vi "Power Driver.vi"(0 "P CH0_curlim, A":dbl=0.08 min=0.01 max=1.0 format="%_6p", 1 "P CH0, V":dbl=3.3000000000000003 min=0.0 max=6.0 format="%_6p", 2 "P CH1_curlim, A":dbl=0.1 min=0.01 max=1.0 format="%_6p", 3 "P CH1_cur, A":dbl=2.0 min=0.0 max=20.0 format="%_6p", 4 "P CH2_curlim, A":dbl=0.01 min=0.01 max=1.0 format="%_6p", 5 "P CH2, V":dbl=-5.0 min=-20.0 max=0.0 format="%_6p", 6 "P CH0":bool, 7 "Instrument Handle In":refnum<k15>, 8 "P CH1":bool, 9 "Error In":errorcluster, 10 "P CH2":bool, 12 "Power OFF":bool) -> (11 "Error Out":errorcluster, 13 "Instrument Handle Out":refnum<k15>, 14 "P CH0_char":dbl(graph)=8.200132019086688e-05, 15 "P CH0_cur, A":dbl=8.200132019086688e-05 format="%_6g", 16 "P CH1_char":dbl(graph)=9.464711192498274e-07, 17 "P CH1_cur, A":dbl=9.464711192498274e-07 format="%_6g", 18 "P CH2_char":dbl(graph)=1.4003158139382402e-06, 19 "P CH2_cur, A":dbl=1.4003158139382402e-06 format="%_6g")   [LabVIEW 2018]
uses:
  <instrlib>/niDCPower/nidcpower.llb/niDCPower Measurement Type.ctl
panel:
  out "Power OFF":bool
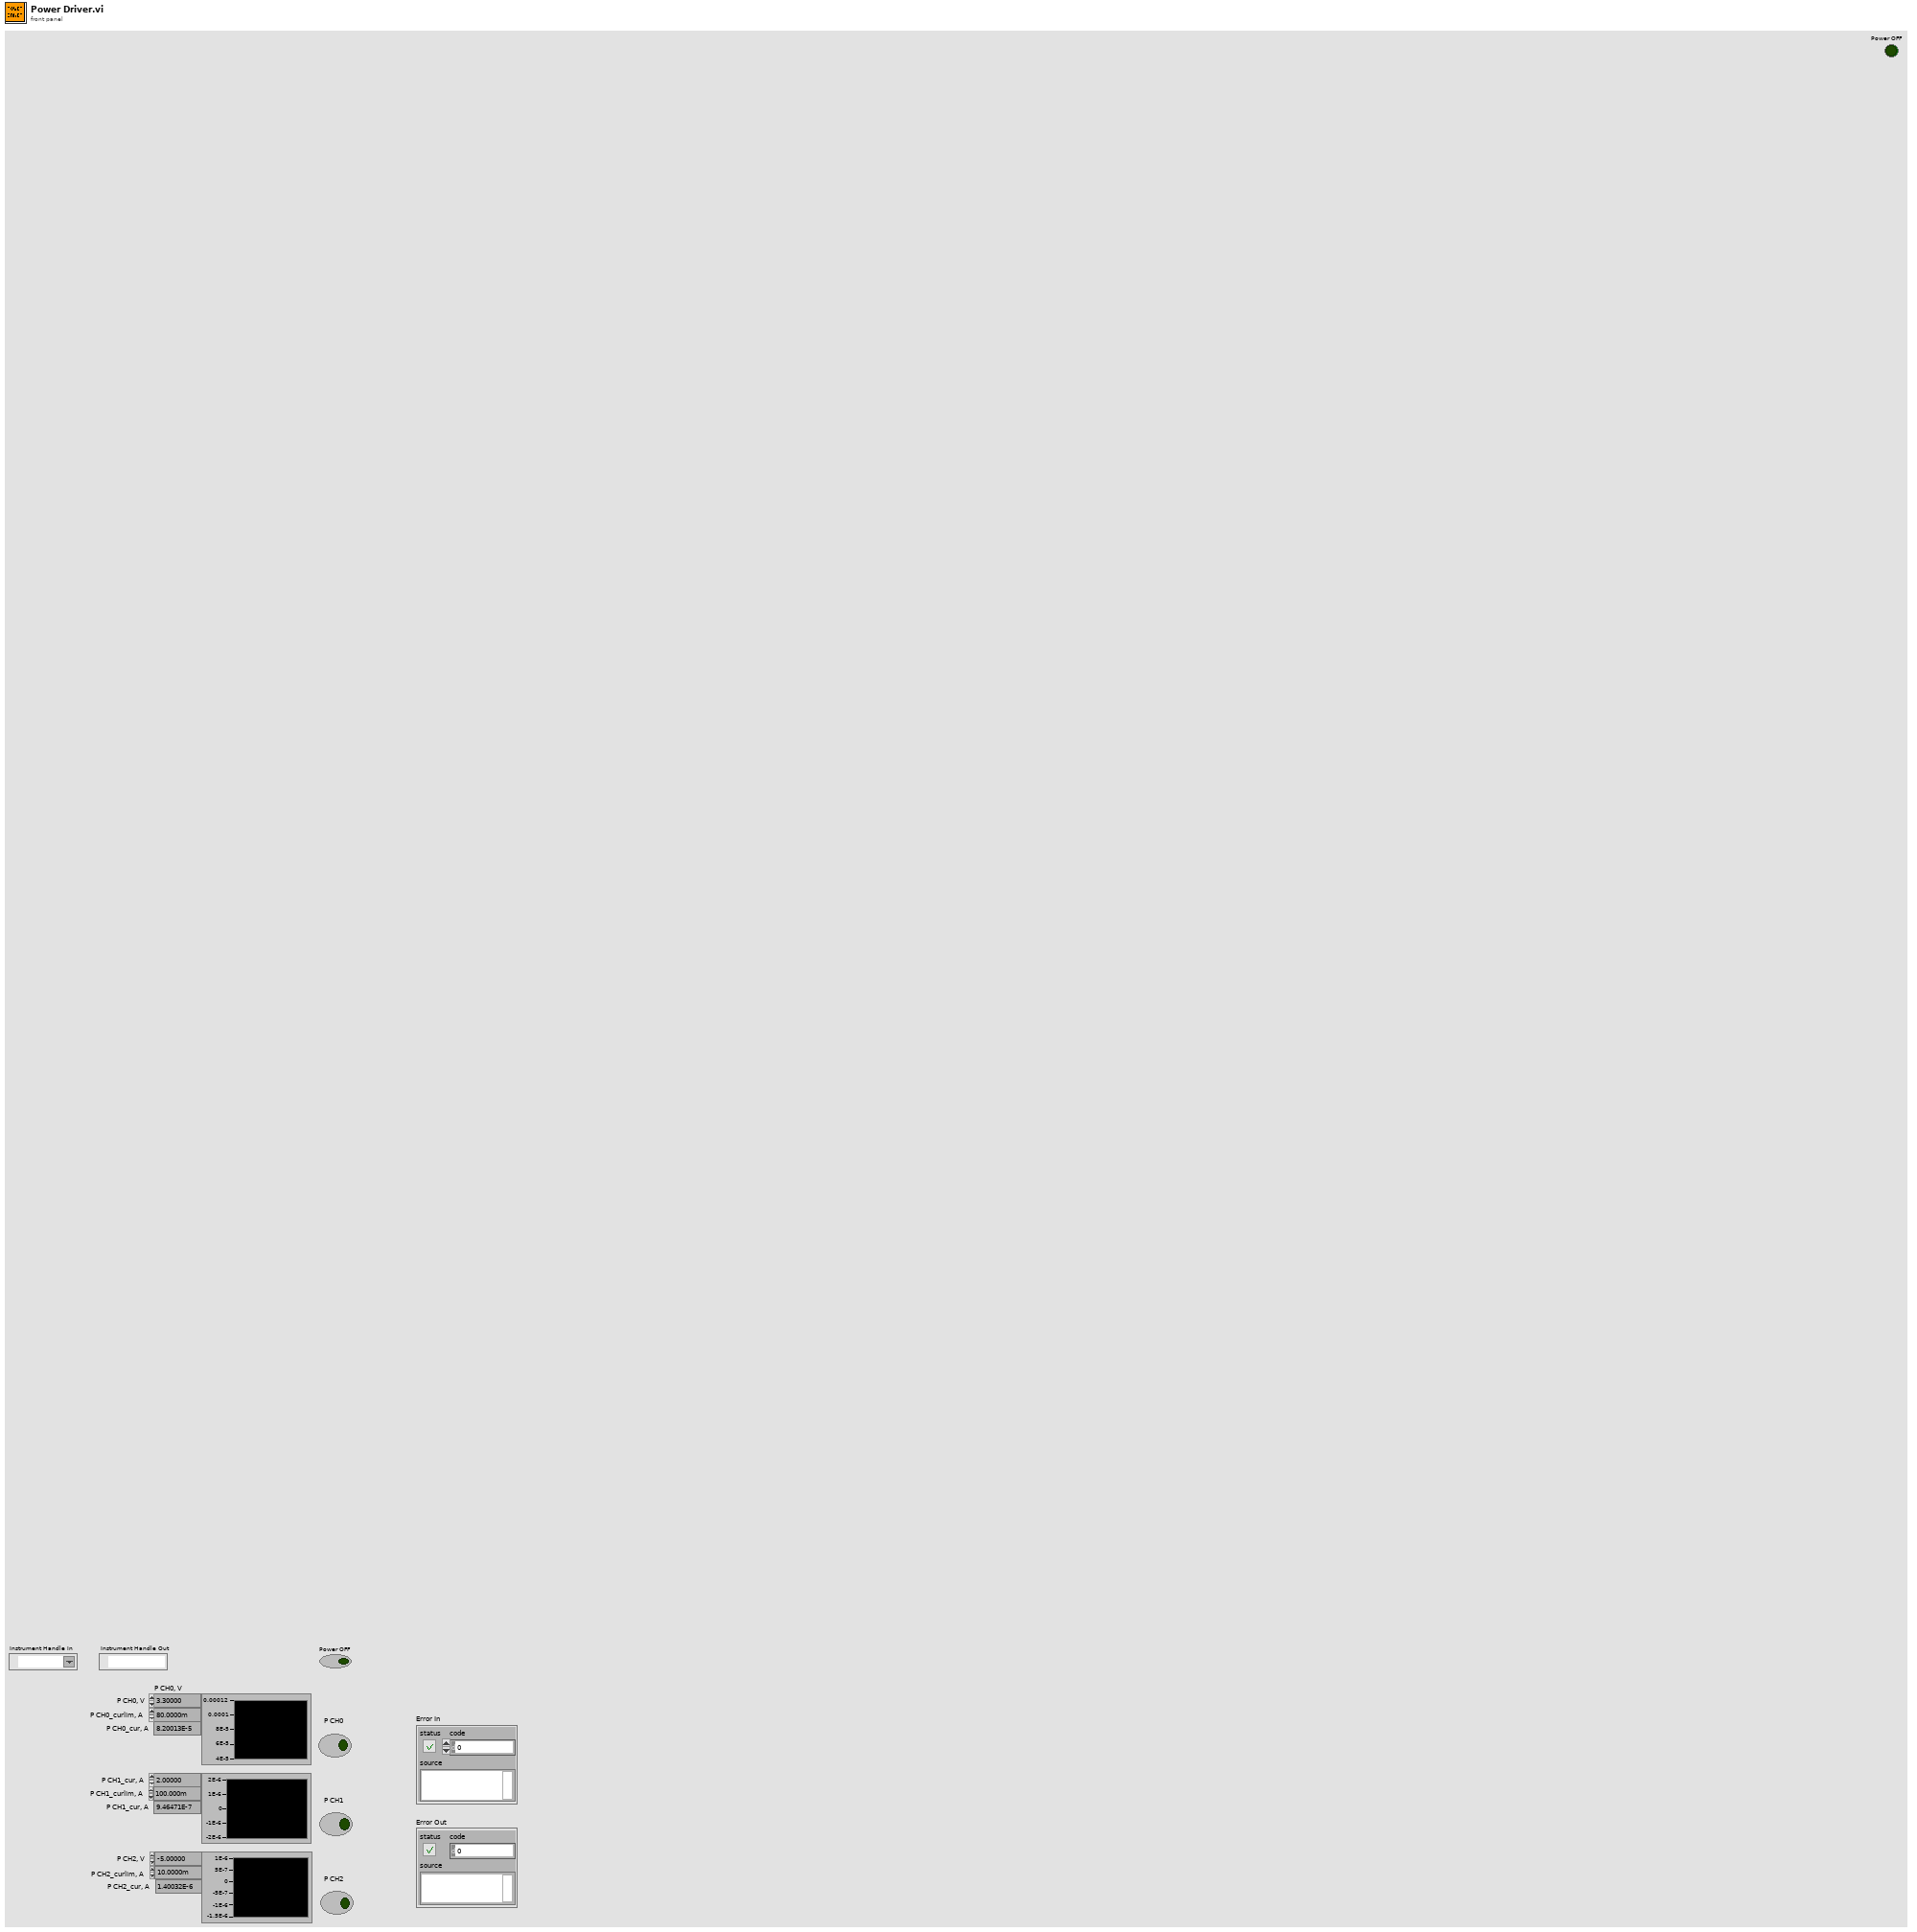
[diagram p1: front panel]
types:
  T1 = typedef "niDCPower Measurement Type.ctl" = i32
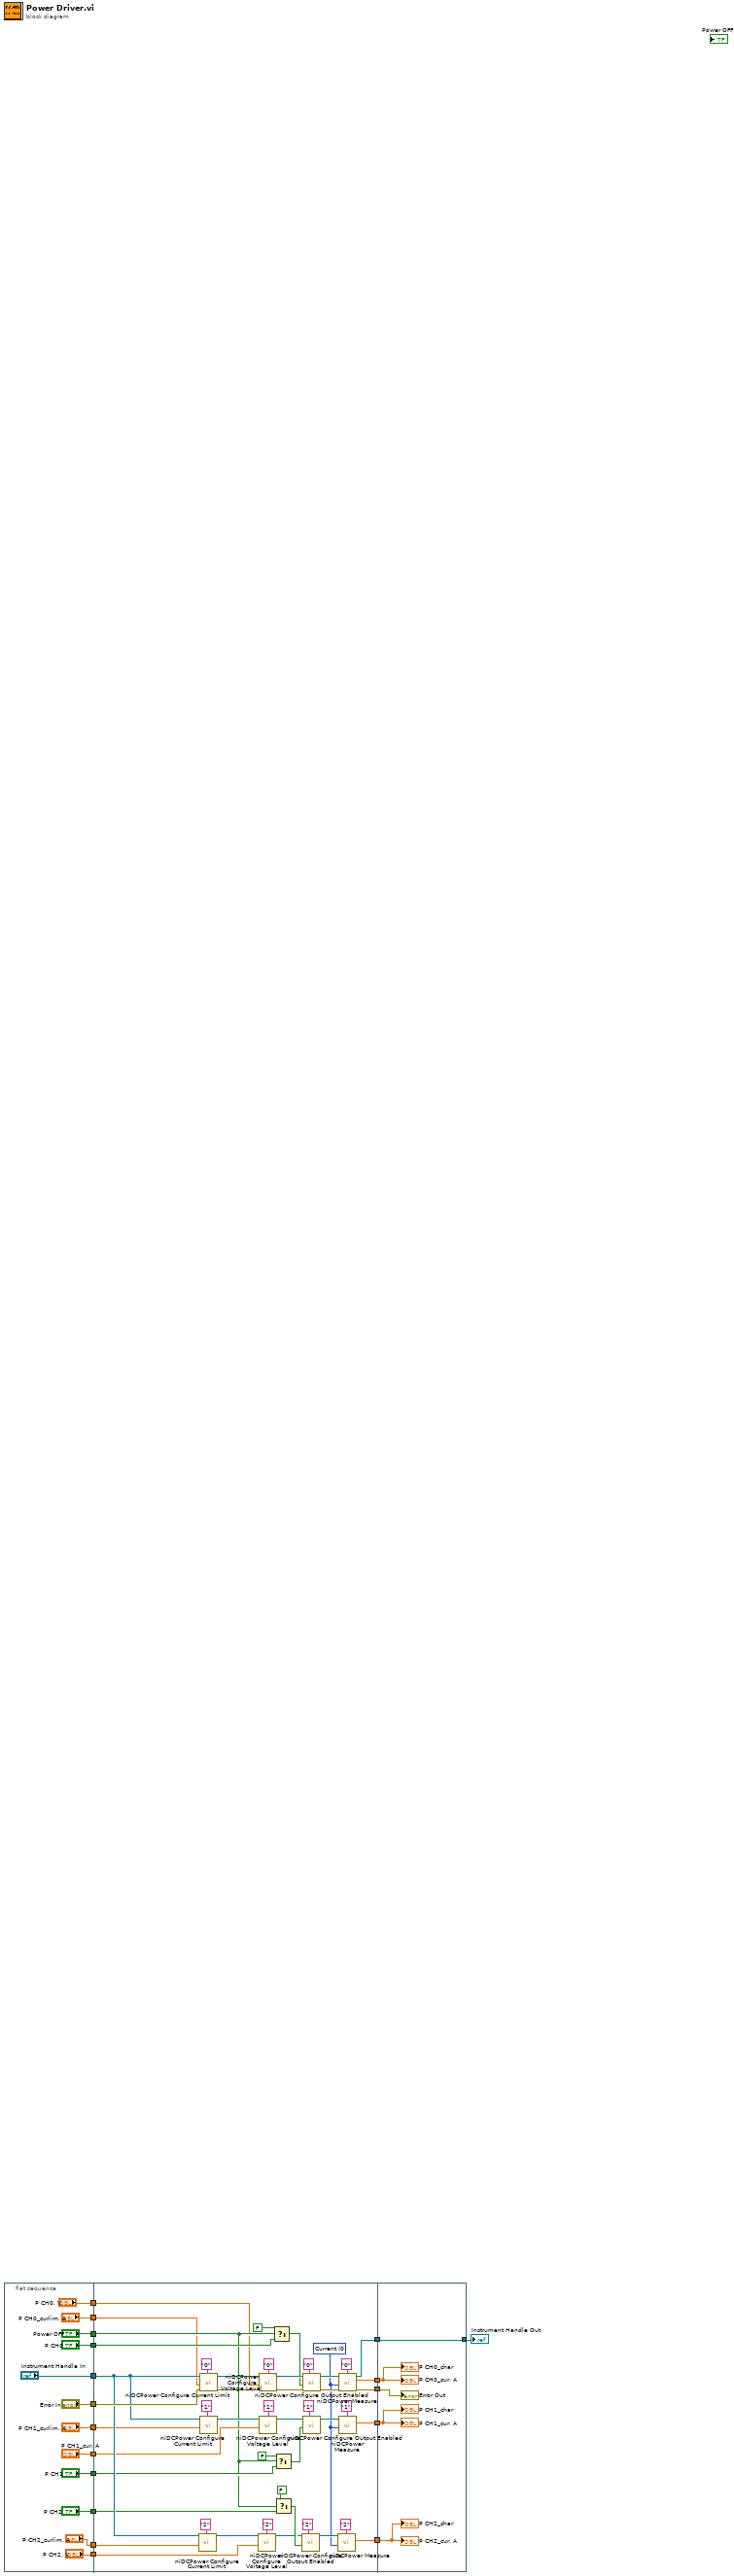
[diagram p0: block diagram]
diagram:
  n1 = flat-sequence {
    tunnel: ["Instrument Handle In"] -> w14
    tunnel: ["Error In"] -> w13
    tunnel: ["P CH1_curlim, A"] -> w12
    tunnel: ["P CH1_cur, A"] -> w11
    tunnel: ["P CH0"] -> w10
    tunnel: ["P CH2"] -> w9
    tunnel: ["P CH1"] -> w8
    tunnel: ["Power OFF"] -> w7
    tunnel: ["P CH2_curlim, A"] -> w6
    tunnel: ["P CH2, V"] -> w5
    tunnel: ["P CH0_curlim, A"] -> w4
    tunnel: ["P CH0, V"] -> w3
    tunnel: [w58] -> w18
    tunnel: [w44] -> w17
    tunnel: [w41] -> w16
    tunnel: [w37] -> w15
    tunnel: w14 -> [w45]
    tunnel: w13 -> [w57]
    tunnel: w12 -> [w43]
    tunnel: w11 -> [w42]
    tunnel: w10 -> [w40]
    tunnel: w9 -> [w39]
    tunnel: w8 -> [w38]
    tunnel: w7 -> [w36]
    tunnel: w6 -> [w35]
    tunnel: w5 -> [w34]
    tunnel: w4 -> [w33]
    tunnel: w3 -> [w32]
    tunnel: [w31] -> w2
    tunnel: w18 -> [w82]
    tunnel: w17 -> [w81]
    tunnel: w16 -> [w83]
    tunnel: w15 -> [w80]
    tunnel: [w79] -> w1
    tunnel: w2 -> [w79]
    frame #0 {
    }
    frame #1 {
      w46 = T1 0 items=["Current", "Voltage"] ("measurement type")
      n2 = call <instrlib>:"niDCPower Configure Current Limit.vi"("current limit"=w35, "channel name"="2", "instrument handle"=w45) -> ("instrument handle out"=w51:refnum<k15>)  [unwired: 7 in, 1 out]
      n3 = call <instrlib>:"niDCPower Configure Current Limit.vi"("error in (no error)"=w57, "current limit"=w33, "channel name"="0", "instrument handle"=w45) -> ("error out"=w56:errorcluster, "instrument handle out"=w72:refnum<k15>)  [unwired: 6 in]
      n4 = call <instrlib>:"niDCPower Configure Current Limit.vi"("current limit"=w43, "channel name"="1", "instrument handle"=w45) -> ("instrument handle out"=w71:refnum<k15>)  [unwired: 7 in, 1 out]
      n5 = call <instrlib>:"niDCPower Configure Voltage Level.vi"("voltage level"=w34, "channel name"="2", "instrument handle"=w51) -> ("instrument handle out"=w52:refnum<k15>)  [unwired: 7 in, 1 out]
      n6 = call <instrlib>:"niDCPower Configure Voltage Level.vi"("error in (no error)"=w56, "voltage level"=w32, "channel name"="0", "instrument handle"=w72) -> ("error out"=w74:errorcluster, "instrument handle out"=w75:refnum<k15>)  [unwired: 6 in]
      n7 = call <instrlib>:"niDCPower Configure Voltage Level.vi"("voltage level"=w42, "channel name"="1", "instrument handle"=w71) -> ("instrument handle out"=w73:refnum<k15>)  [unwired: 7 in, 1 out]
      n8 = Select(t=FALSE, s=w36, f=w40) -> (s? t:f=w59:bool)
      n9 = Select(t=FALSE, s=w36, f=w38) -> (s? t:f=w61:bool)
      n10 = Select(t=FALSE, s=w36, f=w39) -> (s? t:f=w55:bool)
      n11 = call <instrlib>:"niDCPower Configure Output Enabled.vi"("output enabled"=w55, "channel name"="2", "instrument handle"=w52) -> ("instrument handle out"=w53:refnum<k15>)  [unwired: 7 in, 1 out]
      n12 = call <instrlib>:"niDCPower Configure Output Enabled.vi"("error in (no error)"=w74, "output enabled"=w59, "channel name"="0", "instrument handle"=w75) -> ("error out"=w77:errorcluster, "instrument handle out"=w76:refnum<k15>)  [unwired: 6 in]
      n13 = call <instrlib>:"niDCPower Configure Output Enabled.vi"("output enabled"=w61, "channel name"="1", "instrument handle"=w73) -> ("instrument handle out"=w78:refnum<k15>)  [unwired: 7 in, 1 out]
      n14 = call <instrlib>:"niDCPower Measure.vi"("measurement type"=w46, "channel name"="2", "instrument handle"=w53) -> ("measurement"=w37:dbl)  [unwired: 6 in, 2 out]
      n15 = call <instrlib>:"niDCPower Measure.vi"("error in (no error)"=w77, "measurement type"=w46, "channel name"="0", "instrument handle"=w76) -> ("error out"=w58:errorcluster, "measurement"=w41:dbl, "instrument handle out"=w31:refnum<k15>)  [unwired: 5 in]
      n16 = call <instrlib>:"niDCPower Measure.vi"("measurement type"=w46, "channel name"="1", "instrument handle"=w78) -> ("measurement"=w44:dbl)  [unwired: 6 in, 2 out]
    }
    frame #2 {
      "P CH0_char" <- w83
      "P CH0_cur, A" <- w83
      "P CH1_cur, A" <- w81
      "P CH1_char" <- w81
      "P CH2_cur, A" <- w80
      "P CH2_char" <- w80
      "Error Out" <- w82
    }
  }
  "Instrument Handle Out" <- w1
